vi "Remove User.vi"(0 "User Configuration Manager in":refnum<class "User Configuration Manager.lvclass">, 5 "Username":string, 11 "error in (no error)":errorcluster) -> (4 "User Configuration Manager out":refnum<class "User Configuration Manager.lvclass">, 6 "Found":bool, 15 "error out":errorcluster)   [LabVIEW 2019, in "User Configuration Manager.lvlib" / "User Configuration Manager.lvclass"]
uses:
  <vilib>/gpm_packages/@cs/user-manager/Source/User Configuration Manager/User Configuration Manager.lvclass
  <vilib>/gpm_packages/@cs/user-manager/Source/User Configuration Manager/User Configuration Manager.lvclass/User Configuration Manager.ctl
  <vilib>/gpm_packages/@cs/user-manager/Source/User Configuration Manager/Accessors/Read Linked List Ref .vi
  <vilib>/gpm_packages/@cs/linked-list/Source/Linked List/ILinkedList/ILinked List.lvclass
  <vilib>/gpm_packages/@cs/linked-list/Source/Linked List/Linked List Ref/Linked List Ref.lvclass
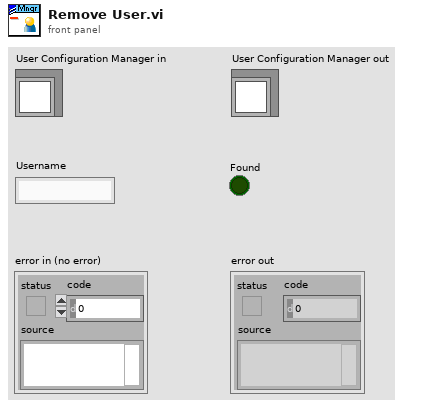
[diagram p1: front panel]
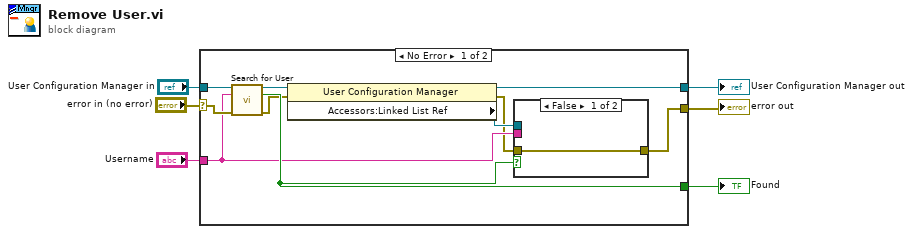
[diagram p0: block diagram]
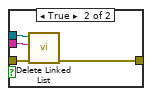
[diagram p2: hidden frame]
diagram:
  n1 = case shown="No Error" "error in (no error)" {
    selector: "error in (no error)" -> [w9 w22]
    tunnel: "User Configuration Manager in" -> [w14 w23]
    tunnel: [w15 w23] -> w5
    tunnel: "Username" -> [w8 _]
    tunnel: [w16 w22] -> w2
    tunnel: [w13 _] -> w1
    frame No Error {
      n2 = call-dynamic "Search for User.vi"("User Configuration Manager in"=w14, "Username"=w8, "error in (no error)"=w9) -> ("User Configuration Manager out"=w11:refnum<class "User Configuration Manager.lvclass">, "Found"=w13:bool, "error out"=w10:errorcluster)  [unwired: 10 in]
      n3 = property class="User Configuration Manager"(reference=w11, error in=w10) -> (reference out=w15:refnum<class "User Configuration Manager.lvclass">, error out=w7:errorcluster, "Accessors:Linked List Ref "=w12:refnum<data-value>)
      n4 = case shown="False" w13 {
        tunnel: [w17 w21] -> w16
        tunnel: w12 -> [_ w20]
        tunnel: w8 -> [_ w19]
        tunnel: w7 -> [w17 w18]
        frame False {
        }
        frame True {
          n5 = call <vilib>:"Delete Linked List.vi"("error in (no error)"=w18, "Linked List ID"=w19, "Linked List Ref"=w20) -> ("error out"=w21:errorcluster)  [unwired: 7 in, 1 out]
        }
      }
    }
    frame Error {
    }
  }
  "error out" <- w2
  "User Configuration Manager out" <- w5
  "Found" <- w1
